vi "sabertooth packetized all motor speeds to all address, command and data.vi"(2 "error in (no error)":errorcluster, 3 "All Motor Speeds":dbl[](array[numeric])=[0.0, 0.0, 0.0, 0.0]) -> (0 "error out":errorcluster, 1 "Data to write":u8[][][](array[numeric]))   [LabVIEW 2018]
uses:
  variables/Sabertooths in use gvar.vi
panel:
  # "Important: this code assumes that in the chain of sabetooths to control, if there is an odd amount of motor speeds being sent, that means that the last\nsabertooth (highest number) is the only one to control one motor. This is important, because this data is not available in the UART message. We only know\nhow many motors to control, and without the rule above, the lonely sabertooth could be anywhere in the mix. This keeps it consistent, without encoding tons\nof data over uart.\n\nThis code also assumes that the array of \"All Motor Speeds\" to be controlled are in increasing order, in increasing motor count. Example: [0.234, -0.345, -0.235, 0.997, 0.456]\n\nThe first two numbers: 0.234, -0.345 are refering to sabertooth 1\n0.234 is \"Motor 1\"\n-0.345 is \"Motor 2\"\n\nand -0.235 and 0.997 are refering to sabertooth 2\n-0.235 is \"Motor 1\"\n0.997 is \"Motor 2\"\n\nsince a saberooth can control only two motors, the next value must go on the third\n0.456 is refering to sabertooth 3, \"Motor 1\""
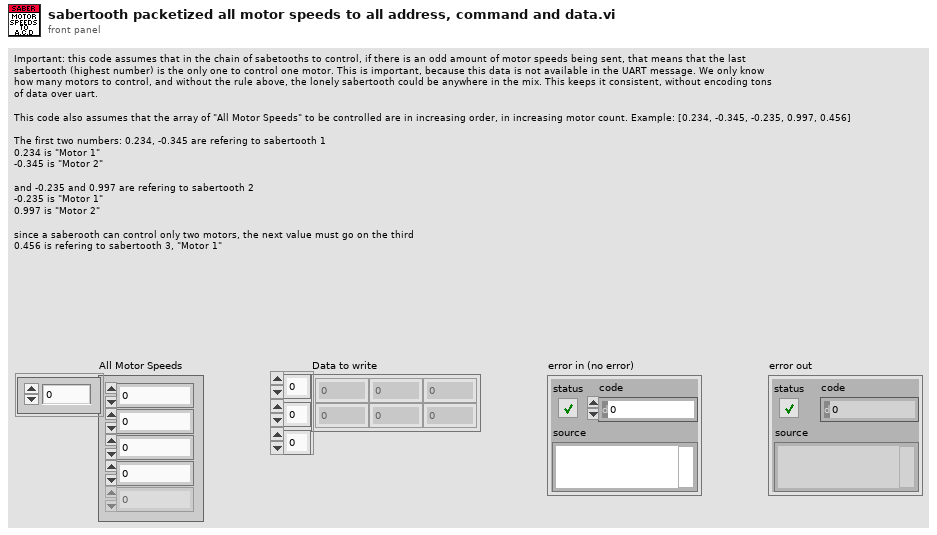
[diagram p1: front panel]
types:
  T1 = typedef "All Addresses.ctl" = u8[]
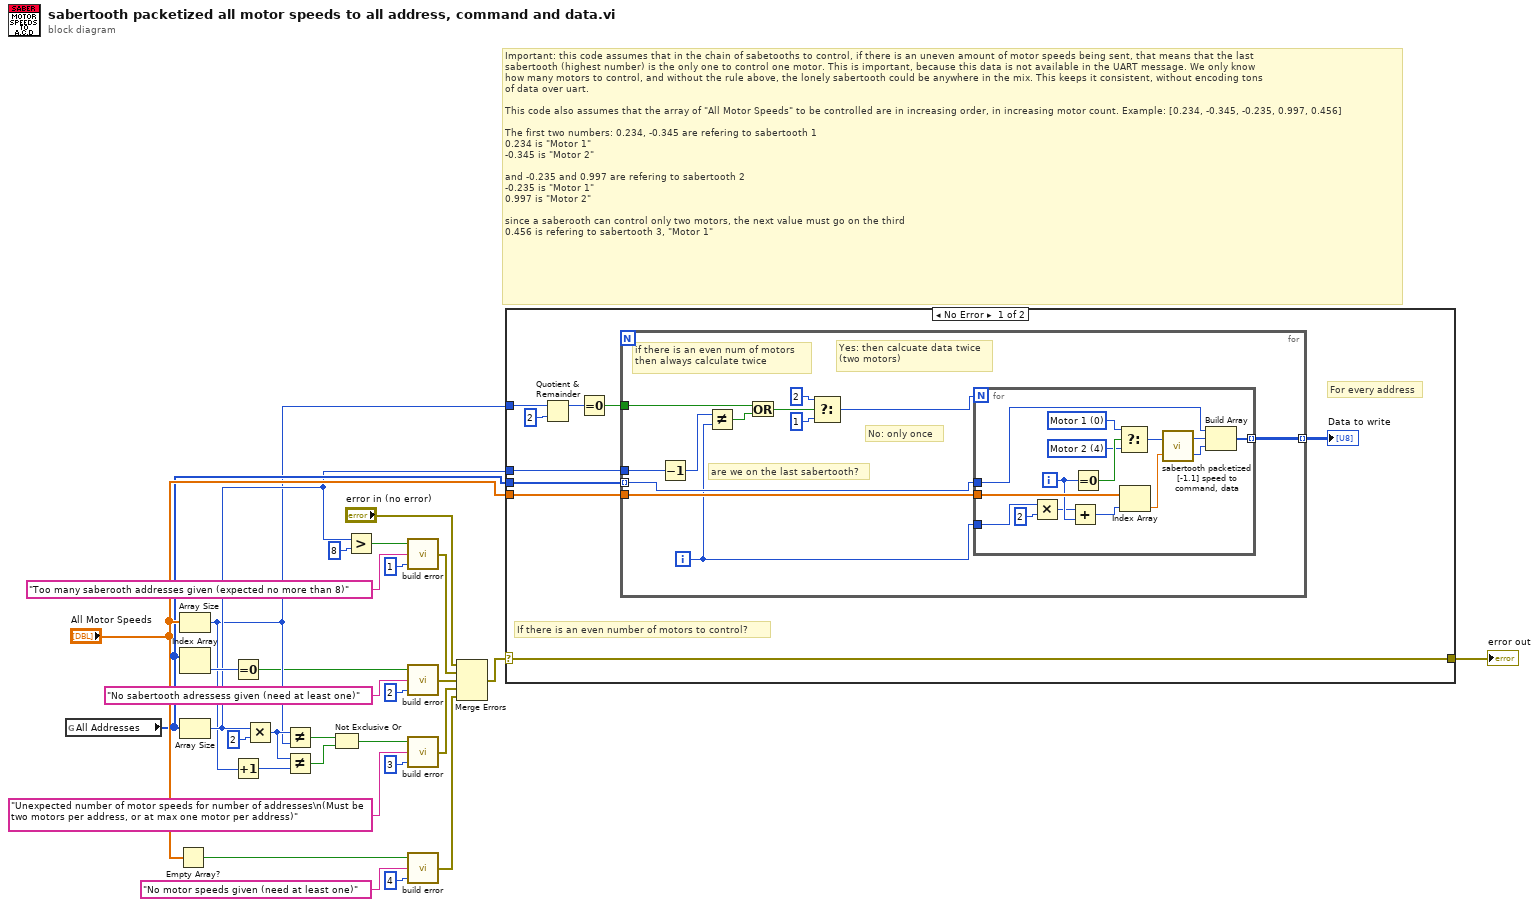
[diagram p0: block diagram]
diagram:
  # "Important: this code assumes that in the chain of sabetooths to control, if there is an uneven amount of motor speeds being sent, that means that the last\nsabertooth (highest number) is the only one to control one motor. This is important, because this data is not available in the UART message. We only know\nhow many motors to control, and without the rule above, the lonely sabertooth could be anywhere in the mix. This keeps it consistent, without encoding tons\nof data over uart.\n\nThis code also assumes that the array of \"All Motor Speeds\" to be controlled are in increasing order, in increasing motor count. Example: [0.234, -0.345, -0.235, 0.997, 0.456]\n\nThe first two numbers: 0.234, -0.345 are refering to sabertooth 1\n0.234 is \"Motor 1\"\n-0.345 is \"Motor 2\"\n\nand -0.235 and 0.997 are refering to sabertooth 2\n-0.235 is \"Motor 1\"\n0.997 is \"Motor 2\"\n\nsince a saberooth can control only two motors, the next value must go on the third\n0.456 is refering to sabertooth 3, \"Motor 1\""
  n1 = global read "Sabertooths in use gvar.vi" "All Addresses"() -> (w25:T1)
  n2 = Empty Array?(array="All Motor Speeds") -> (empty?=w4:bool)
  n3 = Array Size(array="All Motor Speeds") -> (size(s)=w18:i32)
  n4 = Index Array(array=w25) -> (element=w24:u8)  [unwired: 1 in]
  n5 = Array Size(array=w25) -> (size(s)=w19:i32)
  n6 = Equal To 0?(x=w24) -> (x = 0?=w10:bool)
  n7 = Increment(x=w18) -> (x+1=w22:i32)
  n8 = Multiply(x=w19, y=2) -> (x*y=w23:i32)
  n9 = Not Equal?(x=w23, y=w18) -> (x != y?=w20:bool)
  n10 = Not Equal?(x=w23, y=w22) -> (x != y?=w21:bool)
  n11 = Not Exclusive Or(1:w21, 2:w20) -> (0:w6:bool)
  n12 = Greater?(x=w19, y=8) -> (0:w14:bool)
  n13 = call "build error.vi"("Error code"=1 ("code"), "Error msg"="Too many saberooth addresses given (expected no more than 8)" ("source"), "Trigger error"=w14) -> ("error out"=w13:errorcluster)
  n14 = call "build error.vi"("Error code"=2 ("code"), "Error msg"="No sabertooth adressess given (need at least one)" ("source"), "Trigger error"=w10) -> ("error out"=w9:errorcluster)
  n15 = call "build error.vi"("Error code"=3 ("code"), "Error msg"="Unexpected number of motor speeds for number of addresses\n(Must be two motors per address, or at max one motor per address)" ("source"), "Trigger error"=w6) -> ("error out"=w5:errorcluster)
  n16 = call "build error.vi"("Error code"=4 ("code"), "Error msg"="No motor speeds given (need at least one)" ("source"), "Trigger error"=w4) -> ("error out"=w1:errorcluster)
  n17 = Merge Errors("error in (no error)", w13, w9, w5, w1) -> (w26:errorcluster)
  n18 = case shown="No Error" w26 {
    selector: w26 -> [w37 w67]
    tunnel: w25 -> [w39 _]
    tunnel: "All Motor Speeds" -> [w38 _]
    tunnel: [w37 w67] -> w30
    tunnel: w18 -> [w36 _]
    tunnel: w19 -> [w32 _]
    frame No Error {
      # "If there is an even number of motors to control?"
      # "For every address"
      n19 = Quotient & Remainder(x=w36, y=2) -> (x-y*floor(x/y)=w34:i32)  [unwired: 1 out]
      n20 = Equal To 0?(x=w34) -> (x = 0?=w33:bool)
      n21 = for {
        tunnel: w39 -> [w50] mode=indexing
        tunnel: w38 -> [w51]
        tunnel: [w49] -> w31 mode=indexing
        tunnel: w33 -> [w45]
        tunnel: w32 -> [w44]
        i -> [w42]
        # "if there is an even num of motors\nthen always calculate twice"
        # "No: only once"
        # "are we on the last sabertooth?"
        # "Yes: then calcuate data twice\n(two motors)"
        n22 = Decrement(x=w44) -> (x-1=w43:i32)
        n23 = Not Equal?(x=w43, y=w42) -> (x != y?=w41:bool)
        n24 = Or(x=w45, y=w41) -> (x .or. y?=w40:bool)
        n25 = Select(t=2, s=w40, f=1) -> (s? t:f=w46:i32)
        n26 = for {
          N: w46 -> [_]
          tunnel: w51 -> [w58]
          tunnel: w50 -> [w66]
          tunnel: [w59] -> w49 mode=indexing
          tunnel: w42 -> [w55]
          i -> [w56]
          w61 = u8 4 items=["Motor 1"=0, "Motor 2"=4] ("Motor to control")
          w62 = u8 0 items=["Motor 1"=0, "Motor 2"=4] ("Motor to control")
          n27 = Multiply(x=w55, y=2) -> (x*y=w53:i32)
          n28 = Add(x=w53, y=w56) -> (x+y=w52:i32)
          n29 = Equal To 0?(x=w56) -> (x = 0?=w63:bool)
          n30 = Select(t=w62, s=w63, f=w61) -> (s? t:f=w60:u8)
          n31 = Index Array(array=w58, index=w52) -> (element=w57:dbl)
          n32 = call "sabertooth packetized [-1.1] speed to command, data.vi"("Motor speed"=w57, "Motor to control"=w60) -> ("data"=w64:u8, "command"=w65:u8)
          n33 = Build Array(w66, w65, w64) -> (w59:u8[])
        }
      }
      "Data to write" <- w31
    }
    frame Error {
    }
  }
  "error out" <- w30
